vi "Anritsu VNA Restore.vi"(7 "Anritsu VNA":T1, 8 "error in (no error)":errorcluster, 11 "VISA Resource Name":refnum<visa-resource-name>) -> (0 "error out":errorcluster {"code" format="%.0x"}, 3 "dup VISA Resource Name":refnum<visa-resource-name>)   [LabVIEW 2011]
uses:
  TypeDefs/Anritsu VNA Instrument Info.ctl
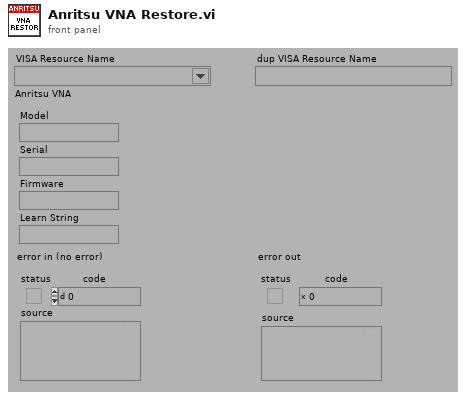
[diagram p1: front panel]
types:
  T1 = typedef "Anritsu VNA Instrument Info.ctl" = cluster{"Model":string, "Serial":string, "Firmware":string, "Learn String":string}
  T2 = typedef "Anritsu VNA Model.ctl" = enum16{"Not Supported", "37XXXX", "MS20XXX", "MS462XX", "MS464XX"}
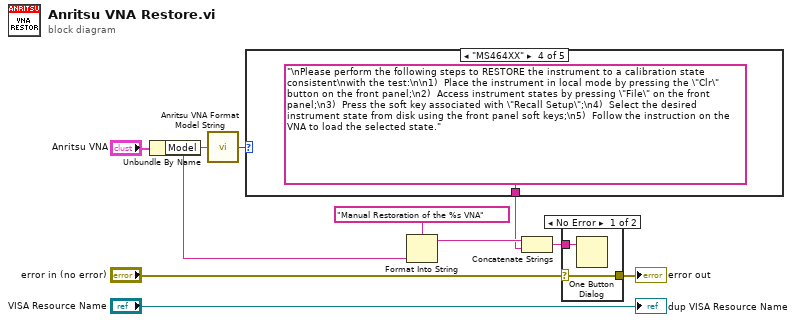
[diagram p0: block diagram]
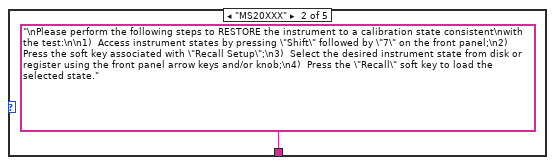
[diagram p3: hidden frame]
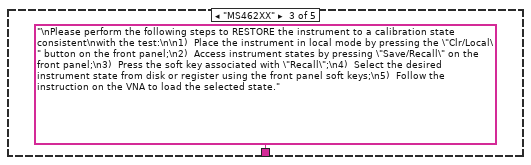
[diagram p4: hidden frame]
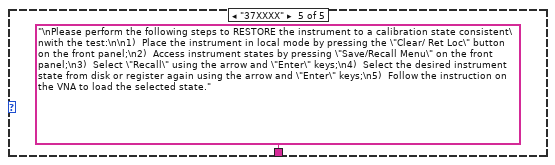
[diagram p5: hidden frame]
diagram:
  n1 = Unbundle By Name("Anritsu VNA") -> ("Model"=w2:string)
  n2 = call "Anritsu VNA Format Model String.vi"("Model"=w2) -> ("Model"=w1:T2)
  n3 = case shown="\"MS464XX\"" w1 {
    tunnel: [_ "\nPlease perform the following steps to RESTORE the instrument to a calibration state consistent\nwith the test:\n\n1)  Access instrument states by pressing \"Shift\" followed by \"7\" on the front panel;\n2)  Press the soft key associated with \"Recall Setup\";\n3)  Select the desired instrument state from disk or register using the front panel arrow keys and/or knob;\n4)  Press the \"Recall\" soft key to load the selected state." "\nPlease perform the following steps to RESTORE the instrument to a calibration state consistent\nwith the test:\n\n1)  Place the instrument in local mode by pressing the \"Clr/Local\" button on the front panel;\n2)  Access instrument states by pressing \"Save/Recall\" on the front panel;\n3)  Press the soft key associated with \"Recall\";\n4)  Select the desired instrument state from disk or register using the front panel soft keys;\n5)  Follow the instruction on the VNA to load the selected state." "\nPlease perform the following steps to RESTORE the instrument to a calibration state consistent\nwith the test:\n\n1)  Place the instrument in local mode by pressing the \"Clr\" button on the front panel;\n2)  Access instrument states by pressing \"File\" on the front panel;\n3)  Press the soft key associated with \"Recall Setup\";\n4)  Select the desired instrument state from disk using the front panel soft keys;\n5)  Follow the instruction on the VNA to load the selected state." "\nPlease perform the following steps to RESTORE the instrument to a calibration state consistent\nwith the test:\n\n1)  Place the instrument in local mode by pressing the \"Clear/ Ret Loc\" button on the front panel;\n2)  Access instrument states by pressing \"Save/Recall Menu\" on the front panel;\n3)  Select \"Recall\" using the arrow and \"Enter\" keys;\n4)  Select the desired instrument state from disk or register again using the arrow and \"Enter\" keys;\n5)  Follow the instruction on the VNA to load the selected state."] -> w7
    frame "Not Supported" {
    }
    frame "MS20XXX" {
    }
    frame "MS462XX" {
    }
    frame "MS464XX" {
    }
    frame "37XXXX" {
    }
  }
  n4 = Format Into String(format string="Manual Restoration of the %s VNA", w2) -> (resulting string=w8:string)  [unwired: 2 in, 1 out]
  n5 = Concatenate Strings(w8, w7) -> (w6:string)
  n6 = case shown="No Error" "error in (no error)" {
    selector: "error in (no error)" -> [w15 w17]
    tunnel: w6 -> [w16 _]
    tunnel: [w15 w17] -> w4
    frame No Error {
      n7 = One Button Dialog(message=w16) -> ()  [unwired: 2 out]
    }
    frame Error {
    }
  }
  "error out" <- w4
  "dup VISA Resource Name" <- "VISA Resource Name"
